vi "2_Speed_Gearbox_AutoShifter.vi"(8 "PhoenixMotorControlDevRef 2":T1={"DeviceStatus"={"status"=FALSE, "code"=0, "source"=""}, "Type"=enum."PWM", "PWM"={"PWM Channel"=enum."Invalid", "DeadBand"={"Name"="", "maxPositivePwm"=0, "minPositivePwm"=0, "centerPwm"=0, "maxNegativePwm"=0, "minNegativePwm"=0, "angularRange"=0}}, "CAN"={"Device Number"=0, "SetOutput VI Ref"=variant(enum8{"Percent VBus", "Current", "Speed", "Position", "Voltage"} enum."Percent VBus"), "GetOutput VI Ref"=variant(refnum<k1> refnum), "Enable VI Ref"=variant(dbl 12.0), "Disable VI Ref"=variant(enum8{"Percent VBus", "Speed", "Position", "Slave", "Unchanged / Invalid", "Voltage Compensation", "Current", "Motion Profile"} enum."Percent VBus"), "Data"=variant}, "Invert"=FALSE, "DIO PWM"={"PWM \"Enable\" Channel"=enum."Invalid", "DIOChannel"=enum."Invalid", "PWM Rate"=0.0}}, 11 "PhoenixMotorControlDevRef":T1={"DeviceStatus"={"status"=FALSE, "code"=0, "source"=""}, "Type"=enum."PWM", "PWM"={"PWM Channel"=enum."Invalid", "DeadBand"={"Name"="", "maxPositivePwm"=0, "minPositivePwm"=0, "centerPwm"=0, "maxNegativePwm"=0, "minNegativePwm"=0, "angularRange"=0}}, "CAN"={"Device Number"=0, "SetOutput VI Ref"=variant(enum8{"Percent VBus", "Current", "Speed", "Position", "Voltage"} enum."Percent VBus"), "GetOutput VI Ref"=variant(refnum<k1> refnum), "Enable VI Ref"=variant(dbl 12.0), "Disable VI Ref"=variant(enum8{"Percent VBus", "Speed", "Position", "Slave", "Unchanged / Invalid", "Voltage Compensation", "Current", "Motion Profile"} enum."Percent VBus"), "Data"=variant}, "Invert"=FALSE, "DIO PWM"={"PWM \"Enable\" Channel"=enum."Invalid", "DIOChannel"=enum."Invalid", "PWM Rate"=0.0}}) -> ()   [LabVIEW 2018]
uses:
  <vilib>/Rock Robotics/WPI/MotorControl/WPI_MotorControlDeviceRef.ctl
  <vilib>/Rock Robotics/WPI/MotorControl/WPI_MotorControlType.ctl
  <vilib>/Rock Robotics/SystemInterfaces/DIO/FPGA_DIOPWMChannel.ctl
  <vilib>/Rock Robotics/WPI/PWM/WPI_PWMDeadband.ctl
  <vilib>/Rock Robotics/SystemInterfaces/DIO/FPGA_DIOChannel.ctl
  <vilib>/Rock Robotics/WPI/Solenoid/WPI_SolenoidValue.ctl
  <vilib>/Rock Robotics/WPI/Solenoid/WPI_SolenoidSetEnum.vi
  <vilib>/Rock Robotics/WPI/ThirdParty/Phoenix-LabVIEW/Motor Controller/Get/CTRE_Phoenix_MotorController_GetQuadratureData.vi
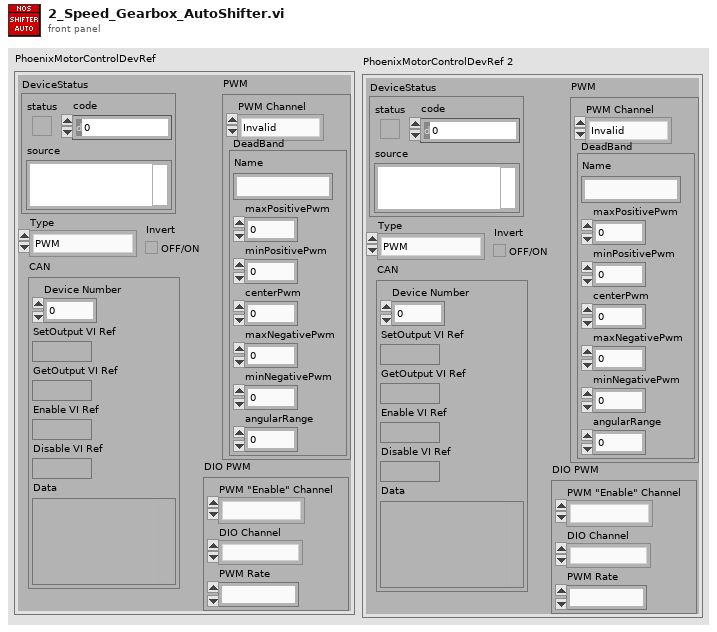
[diagram p1: front panel]
types:
  T1 = typedef "WPI_MotorControlDeviceRef.ctl" = cluster{"DeviceStatus":errorcluster, "Type":T2, "PWM":cluster{"PWM Channel":T3, "DeadBand":T4}, "CAN":cluster{"Device Number":u8, "SetOutput VI Ref":variant, "GetOutput VI Ref":variant, "Enable VI Ref":variant, "Disable VI Ref":variant, "Data":variant}, "Invert":bool, "DIO PWM":cluster{"PWM \"Enable\" Channel":T3, "DIOChannel":T5, "PWM Rate":dbl}}
  T2 = typedef "WPI_MotorControlType.ctl" = enum16{"PWM", "CAN", "DIO PWM"}
  T3 = typedef "FPGA_DIOPWMChannel.ctl" = enum8{"PWM 0", "PWM 1", "PWM 2", "PWM 3", "PWM 4", "PWM 5", "PWM 6", "PWM 7", "PWM 8", "PWM 9", "PWM MXP 0", "PWM MXP 1", "PWM MXP 2", "PWM MXP 3", "PWM MXP 4", "PWM MXP 5", "PWM MXP 6", "PWM MXP 7", "PWM MXP 8", "PWM MXP 9", "Invalid"}
  T4 = typedef "WPI_PWMDeadband.ctl" = cluster{"Name":string, "maxPositivePwm":i32, "minPositivePwm":i32, "centerPwm":i32, "maxNegativePwm":i32, "minNegativePwm":i32, "angularRange":u16}
  T5 = typedef "FPGA_DIOChannel.ctl" = enum8{"DIO 0", "DIO 1", "DIO 2", "DIO 3", "DIO 4", "DIO 5", "DIO 6", "DIO 7", "DIO 8", "DIO 9", "DIO MXP 0", "DIO MXP 1", "DIO MXP 2", "DIO MXP 3", "DIO MXP 4", "DIO MXP 5", "DIO MXP 6", "DIO MXP 7", "DIO MXP 8", "DIO MXP 9", "DIO MXP 10", "DIO MXP 11", "DIO MXP 12", "DIO MXP 13", "DIO MXP 14", "DIO MXP 15", "SPI Port CS1", "SPI Port CS2", "SPI Port CS3", "SPI Port MISO", "SPI Port MOSI", "Invalid"}
  T6 = typedef "WPI_SolenoidValue.ctl" = enum16{"Off", "On", "Forward", "Reverse"}
  T7 = typedef "WPI_SolenoidDevRef.ctl" = cluster{"DevStatus":errorcluster, "Pneumatics Control Module":u8, "Forward Solenoid Channel":T8, "Reverse Solenoid Channel":T8}
  T8 = typedef "WPI_SolenoidChannel.ctl" = enum8{"Solenoid 0", "Solenoid 1", "Solenoid 2", "Solenoid 3", "Solenoid 4", "Solenoid 5", "Solenoid 6", "Solenoid 7", "Invalid"}
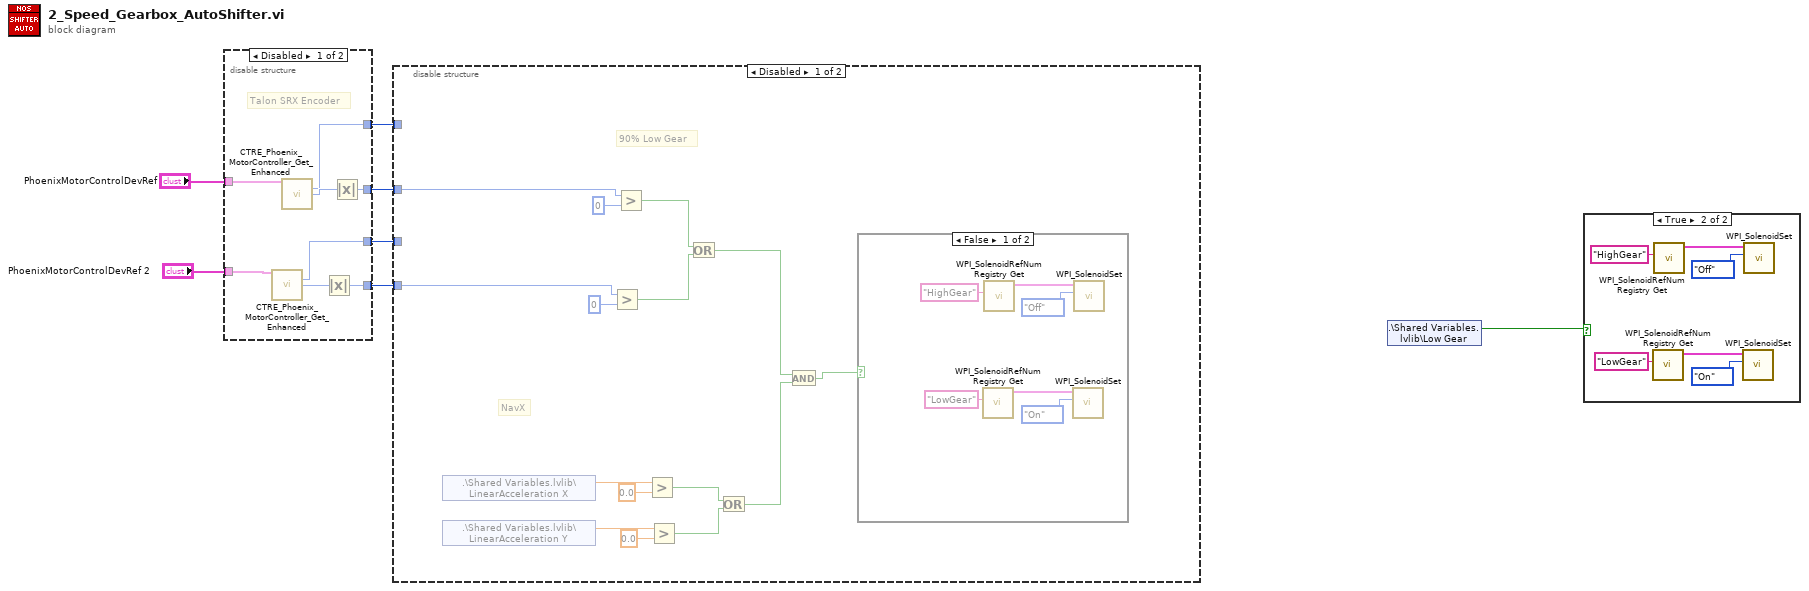
[diagram p0: block diagram]
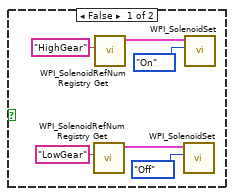
[diagram p3: hidden frame]
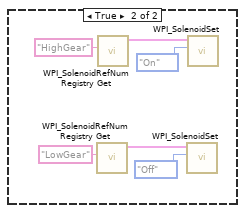
[diagram p4: hidden frame]
diagram:
  n1 = disable-structure shown="Disabled" {
    disable-tunnel: "PhoenixMotorControlDevRef" -> [w15 _]
    disable-tunnel: "PhoenixMotorControlDevRef 2" -> [w14 _]
    disable-tunnel: [w13 _] -> w4
    disable-tunnel: [w10 _] -> w3
    disable-tunnel: [w9 _] -> w2
    disable-tunnel: [w8 _] -> w1
    frame Disabled {
      # "Talon SRX Encoder"
      n2 = call-poly <vilib>:"CTRE_Phoenix_MotorController_Get_Enhanced.vi"("PhoenixMotorControlDevRef"=w14) -> ("Quadrature Position"=w8:i32, "Quadrature Velocity"=w11:i32)  [unwired: 11 in, 2 out]
      n3 = call-poly <vilib>:"CTRE_Phoenix_MotorController_Get_Enhanced.vi"("PhoenixMotorControlDevRef"=w15) -> ("Quadrature Position"=w9:i32, "Quadrature Velocity"=w12:i32)  [unwired: 11 in, 2 out]
      n4 = Absolute Value(x=w11) -> (abs(x)=w10:i32)
      n5 = Absolute Value(x=w12) -> (abs(x)=w13:i32)
    }
    frame Enabled {
    }
  }
  n6 = disable-structure shown="Disabled" {
    disable-tunnel: w4 -> [w17 _]
    disable-tunnel: w3 -> [w16 _]
    disable-tunnel: w2 -> [_ _]
    disable-tunnel: w1 -> [_ _]
    frame Disabled {
      # "NavX"
      # "90% Low Gear"
      n7 = shared-variable ".\\Shared Variables.lvlib\\LinearAcceleration X"() -> (w27:dbl)  [unwired: 1 in, 1 out]
      n8 = shared-variable ".\\Shared Variables.lvlib\\LinearAcceleration Y"() -> (w28:dbl)  [unwired: 1 in, 1 out]
      n9 = Greater?(x=w16, y=0) -> (0:w29:bool)
      n10 = Greater?(x=w17, y=0) -> (0:w30:bool)
      n11 = Greater?(x=w27, y=0.0) -> (0:w26:bool)
      n12 = Greater?(x=w28, y=0.0) -> (0:w25:bool)
      n13 = Or(x=w30, y=w29) -> (x .or. y?=w24:bool)
      n14 = Or(x=w26, y=w25) -> (x .or. y?=w23:bool)
      n15 = And(x=w24, y=w23) -> (x .and. y?=w22:bool)
      n16 = case shown="False" w22 {
        frame False {
          n17 = call <vilib>:"WPI_SolenoidRefNum Registry Get.vi"("refnum name"="LowGear") -> ("SolenoidDevRef"=w34:T7)  [unwired: 9 in, 1 out]
          n18 = call <vilib>:"WPI_SolenoidRefNum Registry Get.vi"("refnum name"="HighGear") -> ("SolenoidDevRef"=w36:T7)  [unwired: 9 in, 1 out]
          n19 = call-poly <vilib>:"WPI_SolenoidSet.vi"("Value"=WPI_SolenoidValue."On", "SolenoidDevRef"=w34) -> ()  [unwired: 8 in, 2 out]
          n20 = call-poly <vilib>:"WPI_SolenoidSet.vi"("Value"=WPI_SolenoidValue."Off", "SolenoidDevRef"=w36) -> ()  [unwired: 8 in, 2 out]
        }
        frame True {
          n21 = call <vilib>:"WPI_SolenoidRefNum Registry Get.vi"("refnum name"="LowGear") -> ("SolenoidDevRef"=w40:T7)  [unwired: 9 in, 1 out]
          n22 = call <vilib>:"WPI_SolenoidRefNum Registry Get.vi"("refnum name"="HighGear") -> ("SolenoidDevRef"=w42:T7)  [unwired: 9 in, 1 out]
          n23 = call-poly <vilib>:"WPI_SolenoidSet.vi"("Value"=WPI_SolenoidValue."Off", "SolenoidDevRef"=w40) -> ()  [unwired: 8 in, 2 out]
          n24 = call-poly <vilib>:"WPI_SolenoidSet.vi"("Value"=WPI_SolenoidValue."On", "SolenoidDevRef"=w42) -> ()  [unwired: 8 in, 2 out]
        }
      }
    }
    frame Enabled {
    }
  }
  n25 = shared-variable ".\\Shared Variables.lvlib\\Low Gear"() -> (w7:bool)  [unwired: 1 in, 1 out]
  n26 = case shown="True" w7 {
    frame False {
      n27 = call <vilib>:"WPI_SolenoidRefNum Registry Get.vi"("refnum name"="LowGear") -> ("SolenoidDevRef"=w46:T7)  [unwired: 9 in, 1 out]
      n28 = call <vilib>:"WPI_SolenoidRefNum Registry Get.vi"("refnum name"="HighGear") -> ("SolenoidDevRef"=w48:T7)  [unwired: 9 in, 1 out]
      n29 = call-poly <vilib>:"WPI_SolenoidSet.vi"("Value"=WPI_SolenoidValue."Off", "SolenoidDevRef"=w46) -> ()  [unwired: 8 in, 2 out]
      n30 = call-poly <vilib>:"WPI_SolenoidSet.vi"("Value"=WPI_SolenoidValue."On", "SolenoidDevRef"=w48) -> ()  [unwired: 8 in, 2 out]
    }
    frame True {
      n31 = call <vilib>:"WPI_SolenoidRefNum Registry Get.vi"("refnum name"="LowGear") -> ("SolenoidDevRef"=w52:T7)  [unwired: 9 in, 1 out]
      n32 = call <vilib>:"WPI_SolenoidRefNum Registry Get.vi"("refnum name"="HighGear") -> ("SolenoidDevRef"=w54:T7)  [unwired: 9 in, 1 out]
      n33 = call-poly <vilib>:"WPI_SolenoidSet.vi"("Value"=WPI_SolenoidValue."On", "SolenoidDevRef"=w52) -> ()  [unwired: 8 in, 2 out]
      n34 = call-poly <vilib>:"WPI_SolenoidSet.vi"("Value"=WPI_SolenoidValue."Off", "SolenoidDevRef"=w54) -> ()  [unwired: 8 in, 2 out]
    }
  }
